vi "SendNotification.vi"(5 "Expiration Date":timestamp=timestamp(3518604913.7528014 s since 1904-01-01) format="%<%x>T", 6 "error in (no error)":errorcluster, 7 "Message":string, 8 "Authentication Token":string="dfed81f65dc0d4d0c684cba4b5c4ef4109437abe", 9 "Channel":string="369unlock") -> (0 "error out":errorcluster)   [LabVIEW 2019]
uses:
  <vilib>/httpClient/POSTBuffer.vi
  <vilib>/httpClient/LabVIEWHTTPClient.lvlib
panel:
  out "body":string="{\"success\": true, \"error_code\": \"\"}"
  out "headers":string="HTTP/1.1 200 OK\r\nServer: nginx/1.4.6 (Ubuntu)\r\nDate: Tue, 07 Jul 2015 14:20:45 GMT\r\nContent-Type: application/json\r\nX-Frame-Options: SAMEORIGIN\r\nAllow: POST, OPTIONS\r\nContent-Length: 35\r\nAccept-Ranges: none\r\nConnection: keep-alive\r\n\r\n"
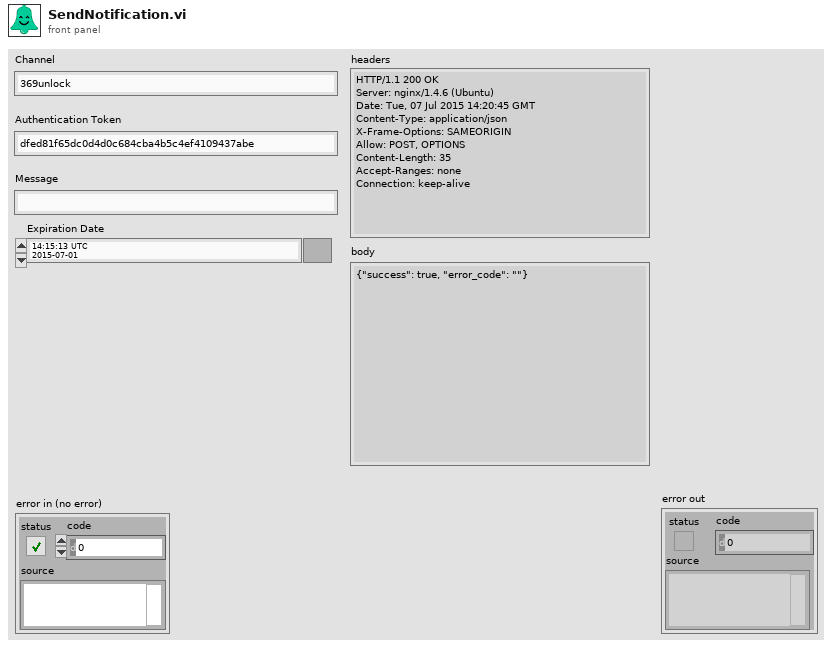
[diagram p1: front panel]
types:
  T1 = typedef "LabVIEWHTTPClient.lvlib/ClientHandle.ctl" = refnum<k1>
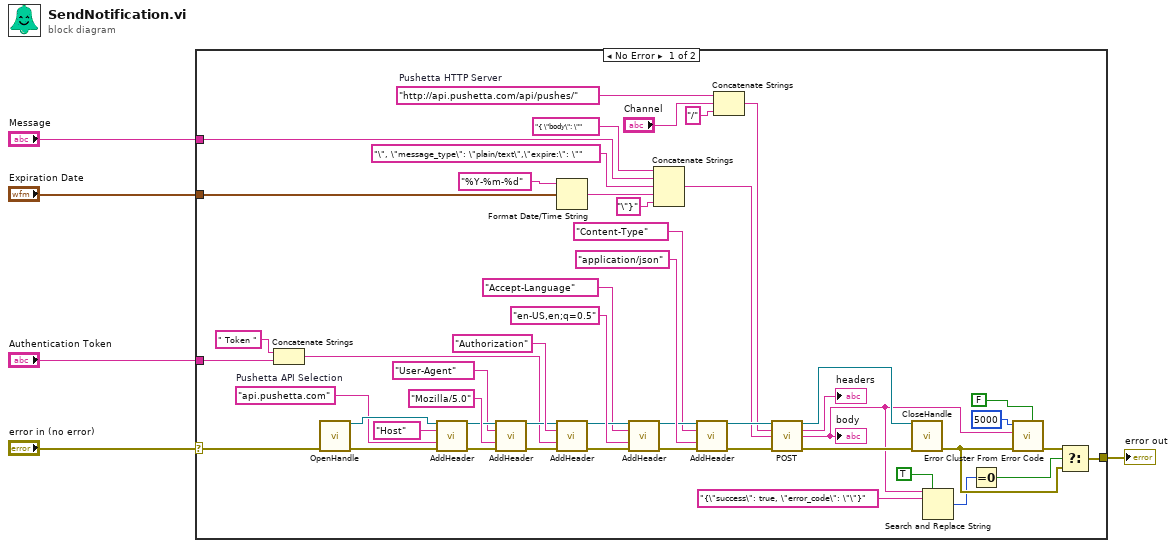
[diagram p0: block diagram]
diagram:
  n1 = case shown="No Error" "error in (no error)" {
    selector: "error in (no error)" -> [w20 w56]
    tunnel: [w12 w56] -> w5
    tunnel: "Authentication Token" -> [w27 _]
    tunnel: "Message" -> [w23 _]
    tunnel: "Expiration Date" -> [w6 _]
    frame No Error {
      w49 = "api.pushetta.com"  # Pushetta API Selection
      w55 = "http://api.pushetta.com/api/pushes/"  # Pushetta HTTP Server
      n2 = Concatenate Strings(" Token " ("string"), w27) -> (w26:string)
      n3 = call <vilib>:"OpenHandle.vi"("error in (no error)"=w20) -> ("client handle out"=w51:T1, "error out"=w50:errorcluster)  [unwired: 13 in]
      n4 = call <vilib>:"AddHeader.vi"("client handle"=w51, "header"="Host", "value"=w49, "error in (no error)"=w50) -> ("client handle out"=w47:T1, "error out"=w46:errorcluster)  [unwired: 10 in]
      n5 = call <vilib>:"AddHeader.vi"("client handle"=w47, "header"="User-Agent", "value"="Mozilla/5.0", "error in (no error)"=w46) -> ("client handle out"=w45:T1, "error out"=w44:errorcluster)  [unwired: 10 in]
      n6 = Format Date/Time String(time format string (%c)="%Y-%m-%d", seconds (now)=w6) -> (date/time string=w8:string)  [unwired: 1 in]
      n7 = call <vilib>:"AddHeader.vi"("client handle"=w45, "header"="Authorization", "value"=w26, "error in (no error)"=w44) -> ("client handle out"=w42:T1, "error out"=w41:errorcluster)  [unwired: 10 in]
      n8 = call <vilib>:"AddHeader.vi"("client handle"=w42, "header"="Accept-Language", "value"="en-US,en;q=0.5", "error in (no error)"=w41) -> ("client handle out"=w39:T1, "error out"=w38:errorcluster)  [unwired: 10 in]
      n9 = Concatenate Strings("{ \"body\": \"" ("string"), w23, "\", \"message_type\": \"plain/text\",\"expire:\": \"" ("string"), w8, "\"}" ("string")) -> (w21:string)
      n10 = call <vilib>:"AddHeader.vi"("client handle"=w39, "header"="Content-Type", "value"="application/json", "error in (no error)"=w38) -> ("client handle out"=w33:T1, "error out"=w29:errorcluster)  [unwired: 10 in]
      n11 = Concatenate Strings(w55, "Channel", "/" ("string")) -> (w30:string)
      n12 = call-poly <vilib>:"POST.vi"("client handle"=w33, "url"=w30, "buffer"=w21, "error in (no error)"=w29) -> ("client handle out"=w32:T1, "headers"=→"headers":string, "body"=w16:string, "error out"=w31:errorcluster)  [unwired: 8 in]
      "body" <- w16
      n13 = call <vilib>:"CloseHandle.vi"("client handle"=w32, "error in (no error)"=w31) -> ("error out"=w15:errorcluster)  [unwired: 13 in]
      n14 = Search and Replace String(replace all?=TRUE ("replace all? (F)"), input string=w16, search string="{\"success\": true, \"error_code\": \"\"}") -> (number of replacements=w10:i32)  [unwired: 5 in, 3 out]
      n15 = Equal To 0?(x=w10) -> (x = 0?=w11:bool)
      n16 = call <vilib>:"Error Cluster From Error Code.vi"("is warning? (False)"=FALSE, "error in (no error)"=w15, "error message (\"\")"=w16, "error code (0)"=5000) -> ("error out"=w14:errorcluster)  [unwired: 5 in]
      n17 = Select(t=w14, s=w11, f=w15) -> (s? t:f=w12:errorcluster)
    }
    frame Error {
    }
  }
  "error out" <- w5
